vi "Read.vi"(8 "error in (no error)":errorcluster caption="entrée d'erreur (pas d'erreur)", 11 "Server TCP_IP (Default) en entrée":refnum<class "Server TCP_IP (Default).lvclass">) -> (0 "error out":errorcluster caption="sortie d'erreur", 3 "Server TCP_IP (Default) en sortie":refnum<class "Server TCP_IP (Default).lvclass">)   [LabVIEW 2020, in "Library Instrument & Equipement.lvlib" / "Library TCP IP.lvlib" / "Server TCP_IP (Default).lvclass"]
uses:
  Server TCP_IP (Default).lvclass
  Server TCP_IP (Default).lvclass/Server TCP_IP (Default).ctl
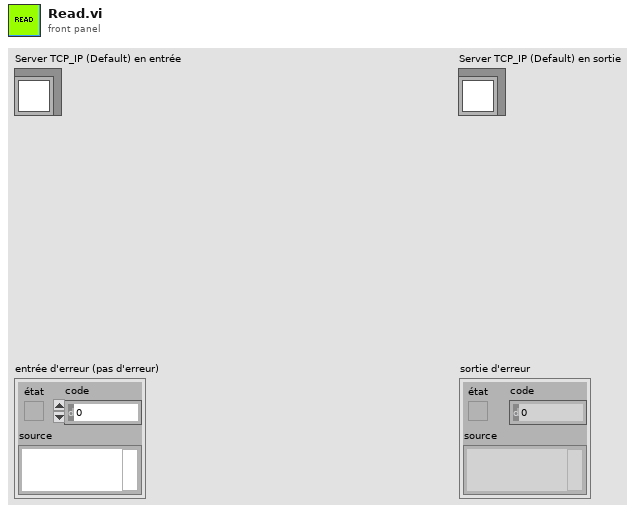
[diagram p1: front panel]
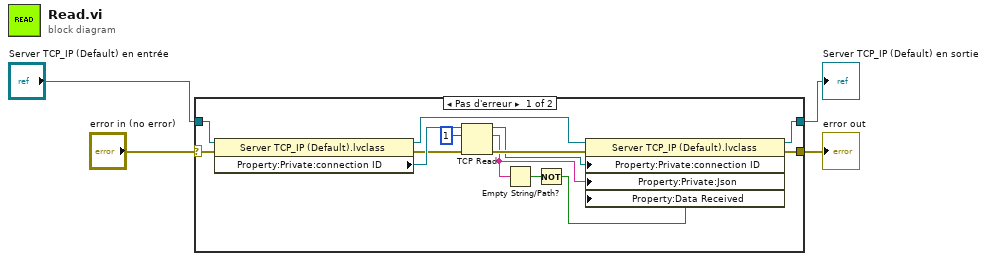
[diagram p0: block diagram]
diagram:
  n1 = case shown="Pas d'erreur" "error in (no error)" {
    selector: "error in (no error)" -> [w11 w19]
    tunnel: [w10 w19] -> w3
    tunnel: [w12 w18] -> w1
    tunnel: "Server TCP_IP (Default) en entrée" -> [w13 w18]
    frame No Error {
      n2 = property class="Server TCP_IP (Default).lvclass"(reference=w13, error in=w11) -> (reference out=w14:refnum<class "Server TCP_IP (Default).lvclass">, error out=w16:errorcluster, "Property:Private:connection ID"=w17:refnum<k5>)
      n3 = TCP Read(connection ID=w17, bytes to read=1 ("octets à lire"), error in (no error)=w16) -> (connection ID out=w6:refnum<k5>, data out=w9:string, error out=w15:errorcluster)  [unwired: 2 in]
      n4 = Empty String/Path?(string/path=w9) -> (empty?=w8:bool)
      n5 = Not(x=w8) -> (.not. x?=w7:bool)
      n6 = property class="Server TCP_IP (Default).lvclass"(reference=w14, error in=w15, "Property:Private:connection ID"=w6, "Property:Private:Json"=w9, "Property:Data Received"=w7) -> (reference out=w12:refnum<class "Server TCP_IP (Default).lvclass">, error out=w10:errorcluster)
    }
    frame Error {
    }
  }
  "error out" <- w3
  "Server TCP_IP (Default) en sortie" <- w1
